vi "8.8.4_다이나믹 이벤트.vi"() -> ()   [LabVIEW 2018]
panel:
  out "문자열":string
  in  "정지":bool
  out "웨이브폼 차트":dbl(graph)
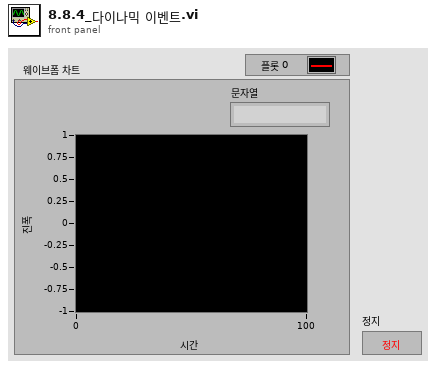
[diagram p1: front panel]
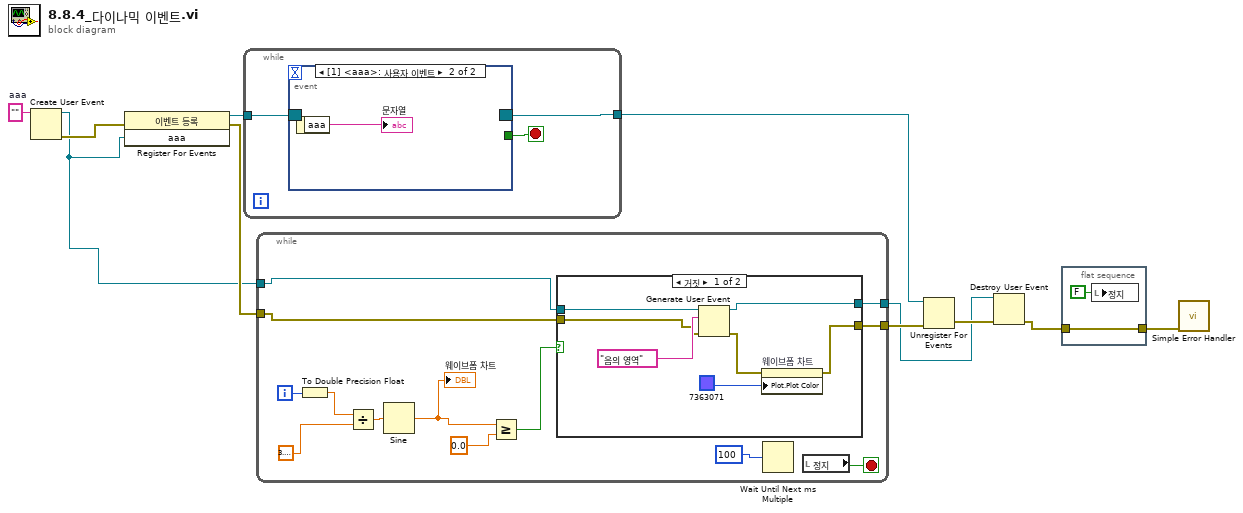
[diagram p0: block diagram]
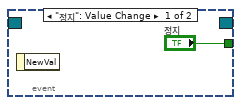
[diagram p2: hidden frame]
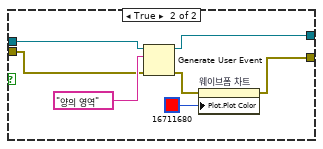
[diagram p3: hidden frame]
diagram:
  w10 = ""  # aaa
  n1 = Create User Event(user event datatype=w10) -> (user event=w1:refnum<user-event>, error out=w11:errorcluster)  [unwired: 1 in]
  n2 = register-events(error in=w11, w1) -> (reference out=w9:refnum<event-registration>, error out=w8:errorcluster)  [unwired: 1 in]
  n3 = while {
    tunnel: w9 -> [w13]
    tunnel: [w12] -> w7
    stop <- w14 stop-if-true
    n4 = event shown="[1] <aaa>: 사용자 이벤트" {
      selector: w13 -> [_ _]
      dyn-events: [_ _] -> w12
      timeout: _ -> [_ _]
      tunnel: ["정지" _] -> w14
      event "정지": Value Change {
        n5 = event-data() -> ()  [unwired: 1 in, 1 out]
      }
      event User Event {
        n6 = event-data() -> ("aaa"=→"문자열":string)  [unwired: 1 in]
      }
    }
  }
  n7 = while {
    tunnel: w1 -> [w20]
    tunnel: w8 -> [w19]
    tunnel: [w18] -> w6
    tunnel: [w17] -> w2
    i -> [w29]
    stop <- w22 stop-if-true
    n8 = To Double Precision Float(number=w29) -> (double precision float=w28:dbl)
    n9 = Divide(x=w28, y=3.141592653589793) -> (x/y=w26:dbl)
    n10 = Sine(x=w26) -> (sin(x)=w23:dbl)
    "웨이브폼 차트" <- w23
    n11 = Greater Or Equal?(x=w23, y=0.0) -> (x >= y?=w21:bool)
    n12 = case shown="거짓" w21 {
      tunnel: w20 -> [w34 w41]
      tunnel: w19 -> [w33 w40]
      tunnel: [w31 w37] -> w18
      tunnel: [w30 w39] -> w17
      frame False {
        n13 = Generate User Event(user event=w34, event data cluster="음의 영역", error in=w33) -> (user event out=w30:refnum<user-event>, error out=w32:errorcluster)  [unwired: 1 in]
        n14 = property on="웨이브폼 차트" class="WFChart (엄격한)"(error in=w32, "Plot.Plot Color"=u32 7363071) -> (error out=w31:errorcluster)  [unwired: 1 in, 1 out]
      }
      frame True {
        n15 = Generate User Event(user event=w41, event data cluster="양의 영역", error in=w40) -> (user event out=w39:refnum<user-event>, error out=w38:errorcluster)  [unwired: 1 in]
        n16 = property on="웨이브폼 차트" class="WFChart (엄격한)"(error in=w38, "Plot.Plot Color"=u32 16711680) -> (error out=w37:errorcluster)  [unwired: 1 in, 1 out]
      }
    }
    n17 = Wait Until Next ms Multiple(millisecond multiple=u32 100 ("ms 배수")) -> ()  [unwired: 1 out]
    n18 = local read "정지"() -> (w22:bool)
  }
  n19 = Unregister For Events(event registration refnum=w7, error in=w6) -> (error out=w5:errorcluster)
  n20 = Destroy User Event(user event=w2, error in=w5) -> (error out=w4:errorcluster)
  n21 = flat-sequence {
    tunnel: w4 -> [w44]
    tunnel: [w44] -> w3
    frame #0 {
      n22 = local write "정지"(FALSE ("정지")) -> ()
    }
  }
  n23 = call <vilib>:"Simple Error Handler.vi"("error in (no error)"=w3) -> ()  [unwired: 4 in, 5 out]
